vi "Customizing Icon and Connector Pane.vi"() -> ()   [LabVIEW 2010]
doc: "This VI demonstrates where to use subVIs to perform repeated calculations."
panel:
  in  "Function 3":cluster{"a":dbl, "b":dbl, "c":dbl, "d":dbl}
  in  "Function 2":cluster{"a":dbl, "b":dbl, "c":dbl, "d":dbl}
  in  "Function 1":cluster{"a":dbl, "b":dbl, "c":dbl, "d":dbl}
  out "XY Graph":cluster{i32[], dbl[]}[](graph)
  in  "Ending x value":i32=100
  in  "Starting x value":i32=-100
  # "ax^3+bx^2+cx+d"
  # "Domain"
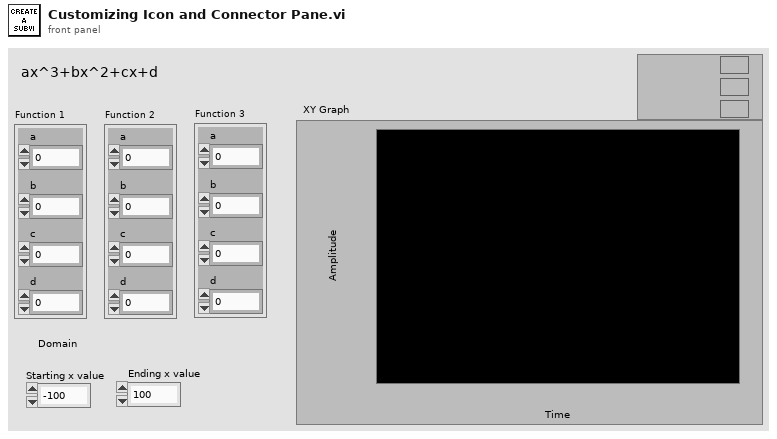
[diagram p1: front panel]
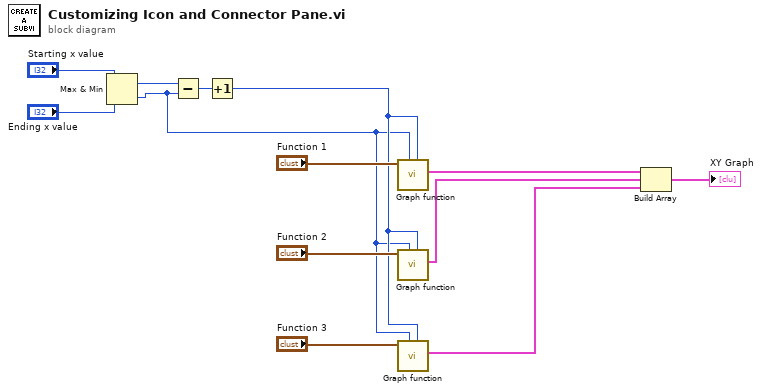
[diagram p0: block diagram]
diagram:
  n1 = Max & Min(x="Starting x value", y="Ending x value") -> (max(x,y)=w11:i32, min(x,y)=w1:i32)
  n2 = Subtract(x=w11, y=w1) -> (x-y=w10:i32)
  n3 = Increment(x=w10) -> (x+1=w2:i32)
  n4 = call "Graph function.vi"("# of iterations"=w2, "Starting x value"=w1, "Function Parameters"="Function 1") -> ("XY Data"=w9:cluster{i32[], dbl[]})  [unwired: 8 in]
  n5 = call "Graph function.vi"("# of iterations"=w2, "Starting x value"=w1, "Function Parameters"="Function 2") -> ("XY Data"=w7:cluster{i32[], dbl[]})  [unwired: 8 in]
  n6 = call "Graph function.vi"("# of iterations"=w2, "Starting x value"=w1, "Function Parameters"="Function 3") -> ("XY Data"=w6:cluster{i32[], dbl[]})  [unwired: 8 in]
  n7 = Build Array(w9, w7, w6) -> (→"XY Graph":cluster{i32[], dbl[]}[])
